vi "BRig_dataCurrent_iTrial.vi"() -> (2 "output_iTrial":i32)   [LabVIEW 2014]
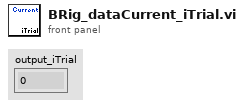
[diagram p1: front panel]
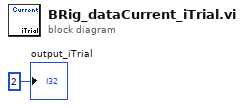
[diagram p0: block diagram]
diagram:
  "output_iTrial" <- 2 ("output_iBlock")
